vi "NinePozwin.vi"(8 "error in (no error)":errorcluster, 10 "Poztion":T1(ring)=enum."中", 11 "VI ref":refnum<vi>) -> (0 "error out":errorcluster, 3 "reference out":refnum<vi>)   [LabVIEW 2017]
panel:
  # "将目标窗口放在屏幕中间，把周围分为9块(3X3),重新设置其相对位置!"
  # "中"
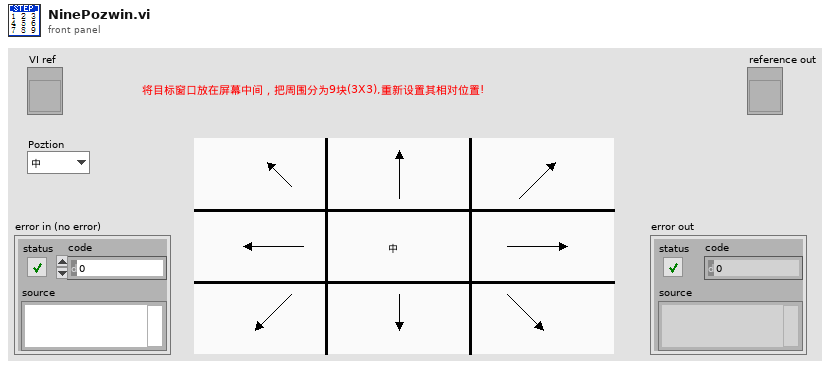
[diagram p1: front panel]
types:
  T1 = enum16{"¨I", "↑", "¨J", "←", "中", "→", "¨L", "↓", "¨K"}
  T2 = typedef "LVRectTypeDef.ctl" = cluster{"Left":i16, "Top":i16, "Right":i16, "Bottom":i16}
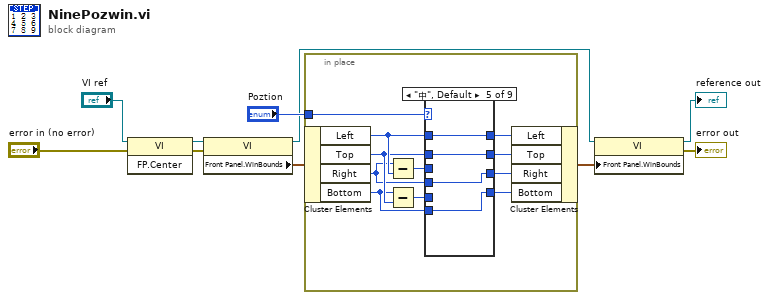
[diagram p0: block diagram]
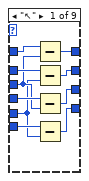
[diagram p2: hidden frame]
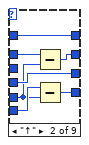
[diagram p3: hidden frame]
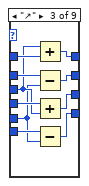
[diagram p4: hidden frame]
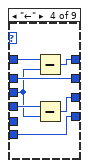
[diagram p5: hidden frame]
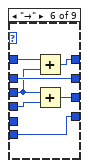
[diagram p6: hidden frame]
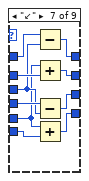
[diagram p7: hidden frame]
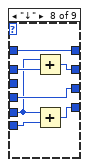
[diagram p8: hidden frame]
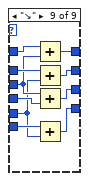
[diagram p9: hidden frame]
diagram:
  n1 = invoke class="VI" method="FP.Center"(reference="VI ref", error in="error in (no error)") -> (reference out=w9:refnum<vi>, error out=w7:errorcluster)  [unwired: 1 in, 1 out]
  n2 = property class="VI"(reference=w9, error in=w7) -> (reference out=w3:refnum<vi>, "Front Panel.WinBounds"=w6:T2)  [unwired: 1 out]
  n3 = in-place {
    in-place-border: "Poztion" -> [w21]
    n4 = in-place-cluster #1(w6) -> ("Left"=w20:i16, "Top"=w19:i16, "Right"=w18:i16, "Bottom"=w17:i16)
    n5 = Subtract(x=w18, y=w20) -> (x-y=w12:i16)
    n6 = Subtract(x=w17, y=w19) -> (x-y=w11:i16)
    n7 = case shown="\"中\", Default" w21 {
      tunnel: w20 -> [w28 w38 w45 w53 w59 w63 w73 w83 w90]
      tunnel: w19 -> [w29 w36 w46 w55 w58 w66 w74 w82 w91]
      tunnel: w18 -> [w30 w37 w47 w51 w57 w64 w75 w81 w92]
      tunnel: w17 -> [w31 w34 w48 w54 w56 w65 w76 w80 w93]
      tunnel: [w27 w38 w44 w52 w59 w62 w72 w83 w89] -> w16
      tunnel: [w26 w35 w41 w55 w58 w66 w69 w79 w88] -> w15
      tunnel: [w25 w37 w43 w50 w57 w61 w71 w81 w87] -> w14
      tunnel: [w24 w33 w40 w54 w56 w65 w68 w78 w86] -> w13
      tunnel: w12 -> [w23 _ w42 w49 _ w60 w70 _ w85]
      tunnel: w11 -> [w22 w32 w39 _ _ _ w67 w77 w84]
      frame "¨I" {
        n8 = Subtract(x=w28, y=w23) -> (x-y=w27:i16)
        n9 = Subtract(x=w29, y=w22) -> (x-y=w26:i16)
        n10 = Subtract(x=w30, y=w23) -> (x-y=w25:i16)
        n11 = Subtract(x=w31, y=w22) -> (x-y=w24:i16)
      }
      frame "↑" {
        n12 = Subtract(x=w36, y=w32) -> (x-y=w35:i16)
        n13 = Subtract(x=w34, y=w32) -> (x-y=w33:i16)
      }
      frame "¨J" {
        n14 = Add(x=w42, y=w45) -> (x+y=w44:i16)
        n15 = Subtract(x=w46, y=w39) -> (x-y=w41:i16)
        n16 = Add(x=w47, y=w42) -> (x+y=w43:i16)
        n17 = Subtract(x=w48, y=w39) -> (x-y=w40:i16)
      }
      frame "←" {
        n18 = Subtract(x=w53, y=w49) -> (x-y=w52:i16)
        n19 = Subtract(x=w51, y=w49) -> (x-y=w50:i16)
      }
      frame "中", Default {
      }
      frame "→" {
        n20 = Add(x=w63, y=w60) -> (x+y=w62:i16)
        n21 = Add(x=w60, y=w64) -> (x+y=w61:i16)
      }
      frame "¨L" {
        n22 = Subtract(x=w73, y=w70) -> (x-y=w72:i16)
        n23 = Add(x=w67, y=w74) -> (x+y=w69:i16)
        n24 = Subtract(x=w75, y=w70) -> (x-y=w71:i16)
        n25 = Add(x=w67, y=w76) -> (x+y=w68:i16)
      }
      frame "↓" {
        n26 = Add(x=w77, y=w82) -> (x+y=w79:i16)
        n27 = Add(x=w77, y=w80) -> (x+y=w78:i16)
      }
      frame "¨K" {
        n28 = Add(x=w90, y=w85) -> (x+y=w89:i16)
        n29 = Add(x=w91, y=w84) -> (x+y=w88:i16)
        n30 = Add(x=w85, y=w92) -> (x+y=w87:i16)
        n31 = Add(x=w93, y=w84) -> (x+y=w86:i16)
      }
    }
    n32 = in-place-cluster #1("Left"=w16, "Top"=w15, "Right"=w14, "Bottom"=w13) -> (w4:T2)
  }
  n33 = property class="VI"(reference=w3, "Front Panel.WinBounds"=w4) -> (reference out=→"reference out":refnum<vi>, error out=→"error out":errorcluster)  [unwired: 1 in]
